vi "Лаба5.vi"() -> ()   [LabVIEW 2019]
uses:
  <vilib>/Utility/file.llb/Read Delimited Spreadsheet (DBL).vi
  <vilib>/Utility/file.llb/Write Delimited Spreadsheet (DBL).vi
panel:
  in  "путь к измененнному файлу":path
  in  "путь к считываему файлу":path
  out "XY Graph":cluster{"all rows":dbl[], "all rows":dbl[]}[](graph)
  out "ток":cluster{i32, i32, "all rows":dbl[]}(graph)
  out "напряжение":cluster{i32, i32, "all rows":dbl[]}(graph)
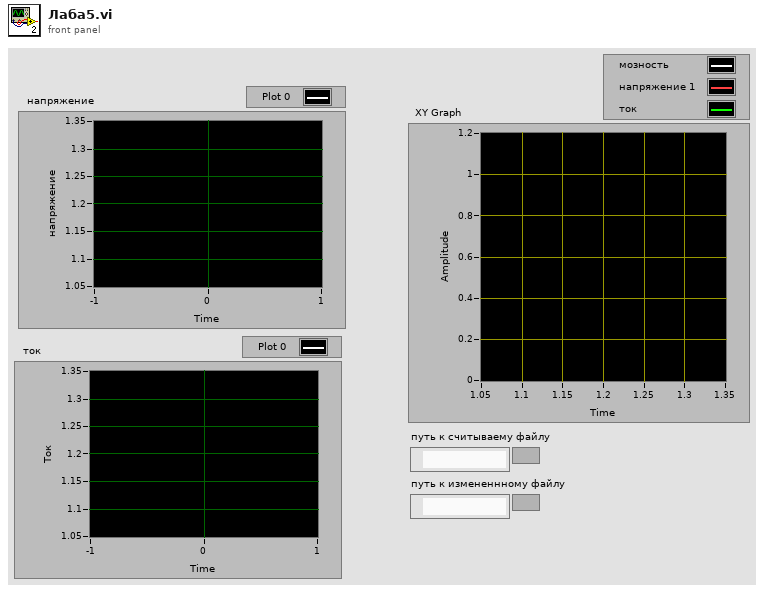
[diagram p1: front panel]
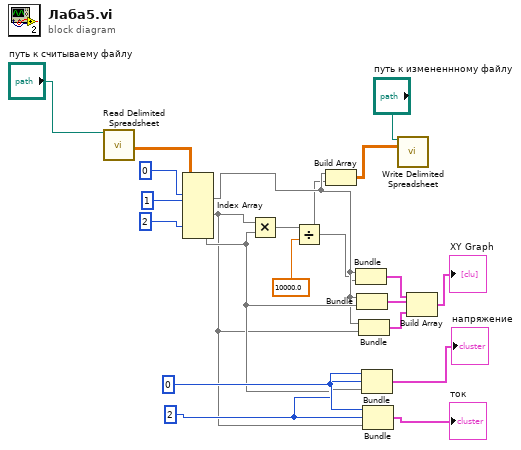
[diagram p0: block diagram]
diagram:
  w11 = 2
  w12 = 0
  n1 = call-poly <vilib>:"Read Delimited Spreadsheet.vi"("file path (dialog if empty)"="путь к считываему файлу") -> ("all rows"=w16:dbl[][])  [unwired: 9 in, 5 out]
  n2 = Index Array(array=w16, index (row) #1=0, index (row) #2=1, index (row) #3=2) -> (element #1=w8:dbl[], element #2=w9:dbl[], element #3=w10:dbl[])  [unwired: 3 in]
  n3 = Multiply(x=w9, y=w10) -> (x*y=w14:dbl[])
  n4 = Divide(x=w14, y=10000.0) -> (x/y=w1:dbl[])
  n5 = Build Array(w8, w1) -> (w15:dbl[][])
  n6 = Bundle("all rows"=w8, w1) -> (w7:cluster{"all rows":dbl[], dbl[]})  [unwired: 1 in]
  n7 = Bundle("all rows"=w8, "all rows"=w10) -> (w6:cluster{"all rows":dbl[], "all rows":dbl[]})  [unwired: 1 in]
  n8 = Bundle("all rows"=w8, "all rows"=w9) -> (w5:cluster{"all rows":dbl[], "all rows":dbl[]})  [unwired: 1 in]
  n9 = Bundle(w12, w11, "all rows"=w10) -> (→"напряжение":cluster{i32, i32, "all rows":dbl[]})  [unwired: 1 in]
  n10 = Bundle(w12, w11, "all rows"=w9) -> (→"ток":cluster{i32, i32, "all rows":dbl[]})  [unwired: 1 in]
  n11 = call-poly <vilib>:"Write Delimited Spreadsheet.vi"("file path (dialog if empty)"="путь к измененнному файлу", "2D data"=w15) -> ()  [unwired: 12 in, 2 out]
  n12 = Build Array(w7, w6, w5) -> (→"XY Graph":cluster{"all rows":dbl[], "all rows":dbl[]}[])
